vi "Global 15 a.vi"() -> ()   [LabVIEW 2025]
panel:
  in  "c":dbl
  in  "b":dbl
  in  "a":dbl
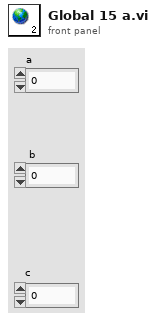
[diagram p1: front panel]
diagram:
